vi "Rec_export one bead XYZ.vi"(10 "beads track":T1 {"centroid"."Y Centroid" format="%.2f"; "centroid"."X Centroid" format="%.2f"; "ROI Des out"."Contours"."Type" items=["No Selection", "Point", "Line", "Rectangle", "Oval", "Polygon", "Freehand Region", "Annulus", "Unused2", "Unused3", "Broken Line", "Freehand Line", "Rotated Rectangle"]}) -> (1 "Z":dbl[](array[numeric]), 2 "Y":dbl[](array[numeric]), 3 "X":dbl[](array[numeric]))   [LabVIEW 2017]
doc: "本VI用来导出某特定球的XYZ数据。"
uses:
  control/Bead track.ctl
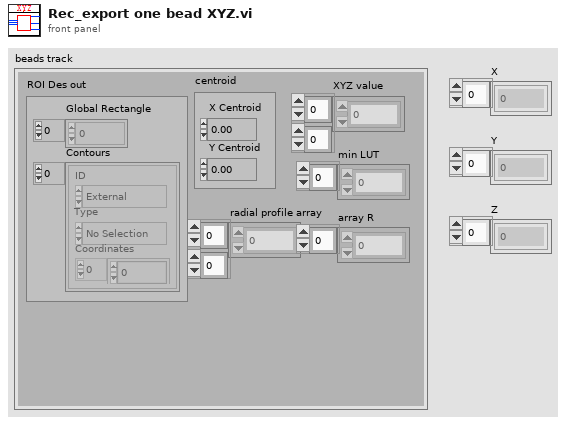
[diagram p1: front panel]
types:
  T1 = typedef "Bead track.ctl" = cluster{"XYZ value":dbl[][], "radial profile array":dbl[][], "min LUT":dbl[], "ROI Des out":T2, "array R":dbl[], "centroid":cluster{"X Centroid":sgl, "Y Centroid":sgl}}
  T2 = typedef "ROI Descriptor" = cluster{"Global Rectangle":i32[], "Contours":cluster{"ID":enum32{"External", "Internal"}, "Type":u32, "Coordinates":i32[]}[]}
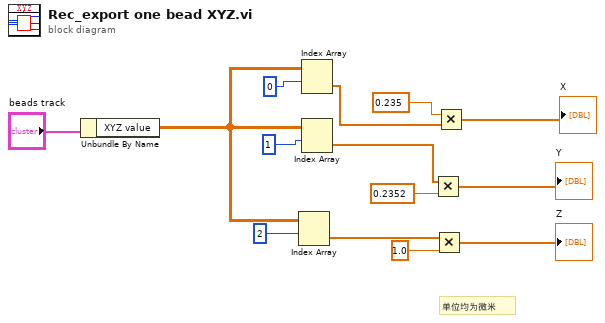
[diagram p0: block diagram]
diagram:
  # "单位均为微米"
  n1 = Unbundle By Name("beads track") -> ("XYZ value"=w5:dbl[][])
  n2 = Index Array(array=w5, index (row)=2 ("禁用的索引 (行)")) -> (element=w11:dbl[])  [unwired: 1 in]
  n3 = Index Array(array=w5, index (row)=0 ("禁用的索引 (行)")) -> (element=w9:dbl[])  [unwired: 1 in]
  n4 = Index Array(array=w5, index (row)=1 ("禁用的索引 (行)")) -> (element=w10:dbl[])  [unwired: 1 in]
  n5 = Multiply(x=w10, y=0.2352) -> (x*y=→"Y":dbl[])
  n6 = Multiply(x=w11, y=1.0) -> (x*y=→"Z":dbl[])
  n7 = Multiply(x=0.235, y=w9) -> (x*y=→"X":dbl[])
